vi "Setup Statically-Linked subWorkers.vi"(8 "error in":errorcluster, 11 "MainUI in":refnum<class "MainUI.lvclass">) -> (0 "error out":errorcluster, 3 "MainUI out":refnum<class "MainUI.lvclass">)   [LabVIEW 2019, in "MainUI.lvclass"]
doc: "This VI performs a setup of all the statically-linked subWorkers that belong to the Worker that owns this VI. This VI must be called <b>before</b> any statically-linked subWorkers are called."
uses:
  MainUI.lvclass
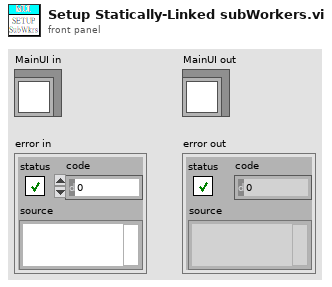
[diagram p1: front panel]
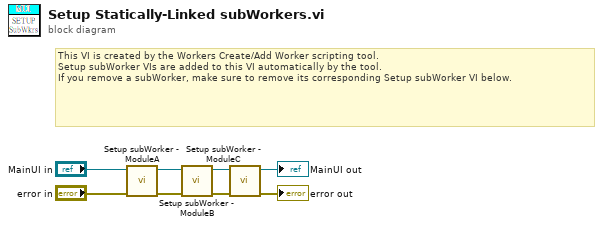
[diagram p0: block diagram]
diagram:
  # "This VI is created by the Workers Create/Add Worker scripting tool.\nSetup subWorker VIs are added to this VI automatically by the tool.\nIf you remove a subWorker, make sure to remove its corresponding Setup subWorker VI below."
  n1 = call "Setup subWorker - ModuleA.vi"("error in"="error in", "MainUI in"="MainUI in") -> ("error out"=w7:errorcluster, "MainUI out"=w4:refnum<class "MainUI.lvclass">)  [unwired: 8 in]
  n2 = call "Setup subWorker - ModuleB.vi"("error in"=w7, "MainUI in"=w4) -> ("error out"=w5:errorcluster, "MainUI out"=w2:refnum<class "MainUI.lvclass">)  [unwired: 8 in]
  n3 = call "Setup subWorker - ModuleC.vi"("error in"=w5, "MainUI in"=w2) -> ("error out"=→"error out":errorcluster, "MainUI out"=→"MainUI out":refnum<class "MainUI.lvclass">)  [unwired: 8 in]
